vi "Clear Unsaved Changes.vi"(11 "ConfigManager.Text in":refnum<class "ConfigManager.Text.lvclass">) -> (3 "ConfigManager.Text out":refnum<class "ConfigManager.Text.lvclass">)   [LabVIEW 2013, in "CfgManager.Text.lvlib" / "ConfigManager.Text.lvclass"]
uses:
  ConfigManager.Text.lvclass
  ConfigManager.Text.lvclass/ConfigManager.Text.ctl
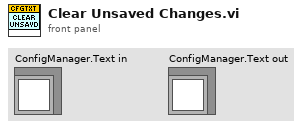
[diagram p1: front panel]
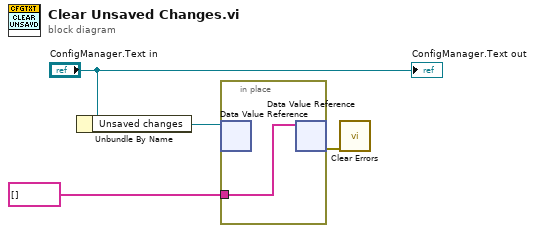
[diagram p0: block diagram]
diagram:
  n1 = Unbundle By Name("ConfigManager.Text in") -> ("Unsaved changes"=w4:refnum<data-value>)
  n2 = in-place {
    in-place-border: string[] [] ("Unsaved changes") -> [w5]
    n3 = in-place-dvr #1(w4) -> ()  [unwired: 2 out]
    n4 = in-place-dvr #1(w5) -> (w1:errorcluster)  [unwired: 1 out]
  }
  n5 = call <vilib>:"Clear Errors.vi"("error in (no error)"=w1) -> ()  [unwired: 6 in, 1 out]
  "ConfigManager.Text out" <- "ConfigManager.Text in"
